vi "Turn On-Off 5V.vi"(8 "error in (no error)":errorcluster, 10 "Value":bool=TRUE, 11 "I-O in":refnum<class "Copy of I-O.lvclass">) -> (0 "error out":errorcluster, 3 "I-O out":refnum<class "Copy of I-O.lvclass">)   [LabVIEW 2016]
uses:
  Copy of I-O.lvclass
panel:
  out "5V":i32
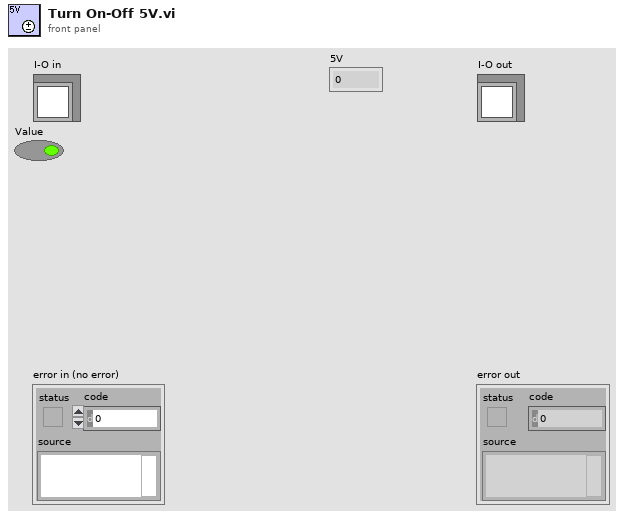
[diagram p1: front panel]
types:
  T1 = typedef "Copy of I-O.lvclass/Pin Map.ctl" = cluster{"Region Valves":i32[], "Extra Valves":dbl[][], "Tool Primary Valve":i32, "Tool Secondary Valve":i32, "Region Sensors":i32[], "Extra Sensors":dbl[][], "Tool Primary Sensor":dbl, "Tool Secondary Sensor":dbl, "Compression Sensor":dbl, "5V":i32, "NTU_Glue":dbl}
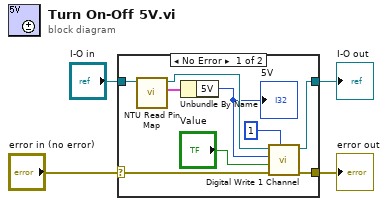
[diagram p0: block diagram]
diagram:
  n1 = case shown="No Error" "error in (no error)" {
    selector: "error in (no error)" -> [w12 w15]
    tunnel: [w11 w15] -> w3
    tunnel: [w13 w14] -> w1
    tunnel: "I-O in" -> [w5 w14]
    frame No Error {
      n2 = call-dynamic "NTU Read Pin Map.vi"("I-O in"=w5) -> ("Pin Map"=w8:T1, "I-O out"=w7:refnum<class "Copy of I-O.lvclass">)  [unwired: 8 in, 1 out]
      n3 = Unbundle By Name(w8) -> ("5V"=w6:i32)
      "5V" <- w6
      n4 = call-dynamic "Digital Write 1 Channel.vi"("DAQ Module"=1, "error constant"=w12, "Value"="Value", "Channel"=w6, "I-O.lvclass"=w7) -> ("error IO"=w11:errorcluster, "I-O.lvclass 2"=w13:refnum<class "Copy of I-O.lvclass">)  [unwired: 5 in]
    }
    frame Error {
    }
  }
  "error out" <- w3
  "I-O out" <- w1
